vi "add scan position(SubVI).vi"(10 "字符串":string) -> (0 "布尔 3":bool, 2 "连接的字符串":string)   [LabVIEW 2019, in "SubVI.lvlib"]
uses:
  SubVI.lvlib
panel:
  in  "Number of Step":i32=2
  in  "Step Delay(secs)":dbl
  in  "Increments":dbl=10.0
  in  "cancel":bool
  in  "ok":bool
  in  "Approach":i32(ring)=1 items=["Pause", "Sweep"]
  in  "Speed":i32 min=0 max=14
  in  "Final Position":dbl min=-140000.0 max=140000.0
  in  "Initial Position":dbl min=-140000.0 max=140000.0
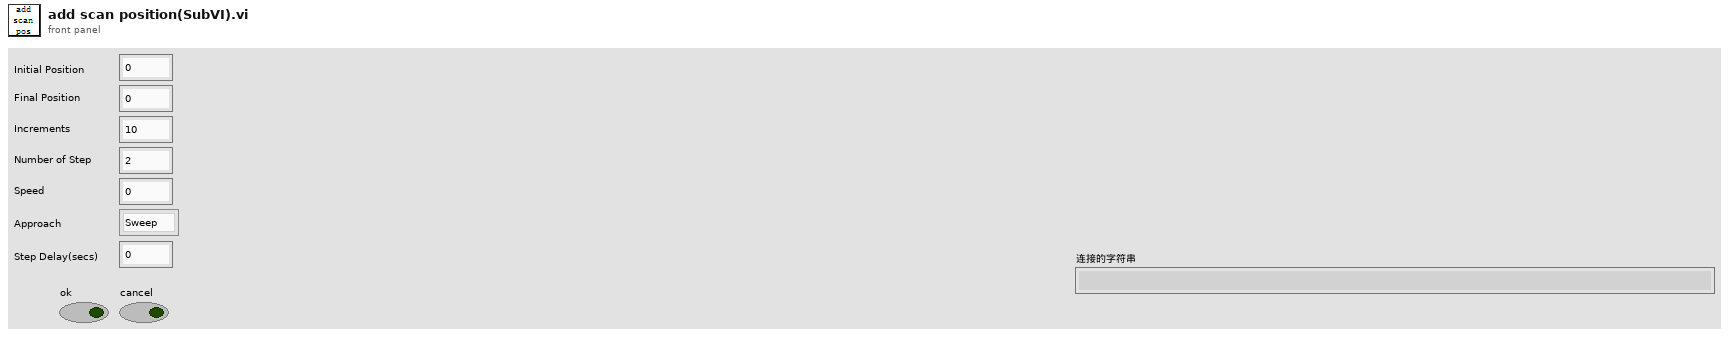
[diagram p1: front panel]
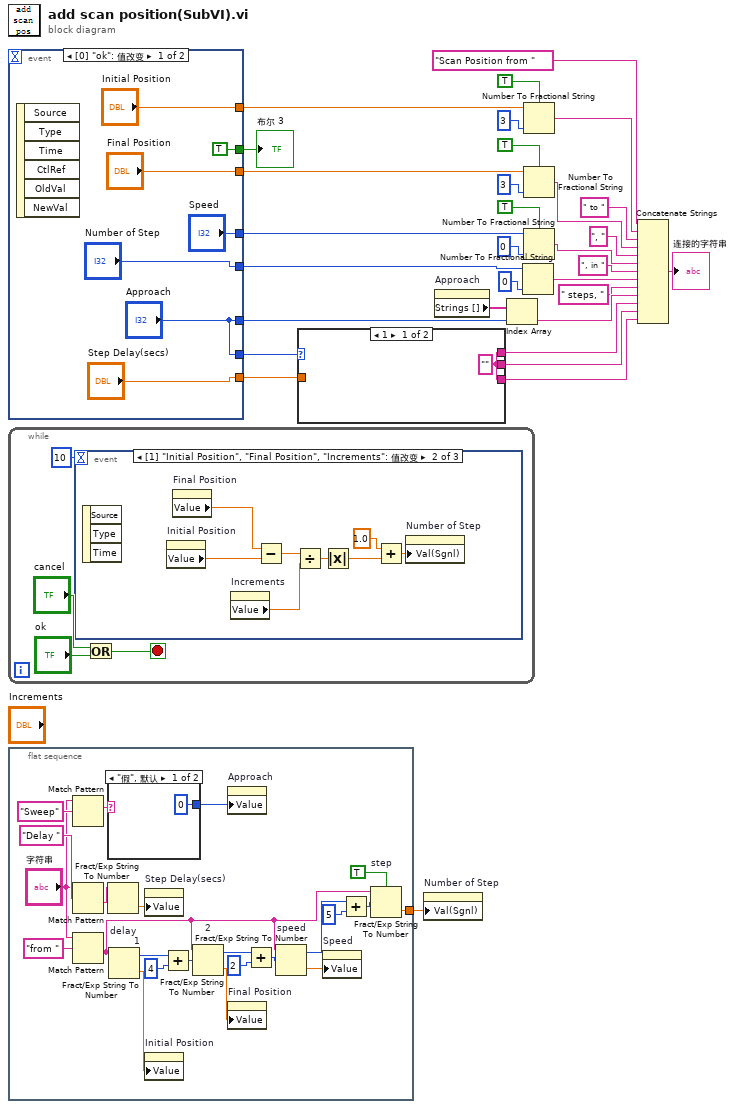
[diagram p0: block diagram]
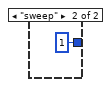
[diagram p2: hidden frame]
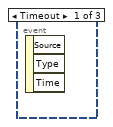
[diagram p3: hidden frame]
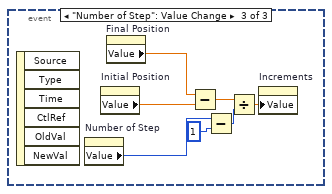
[diagram p4: hidden frame]
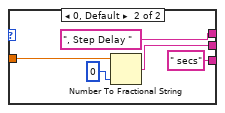
[diagram p5: hidden frame]
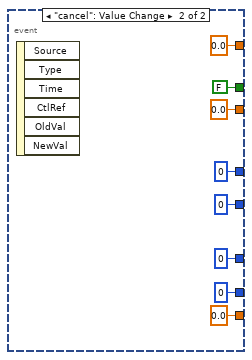
[diagram p6: hidden frame]
diagram:
  n1 = event shown="[0] \"ok\": 值改变" {
    selector: _ -> [_ _]
    dyn-events: _ -> [_ _]
    timeout: _ -> [_ _]
    tunnel: ["Final Position" 0.0 ("Field 2")] -> w20
    tunnel: ["Speed" 0 ("Rate输入")] -> w17
    tunnel: ["Initial Position" 0.0 ("Field")] -> w29
    tunnel: [TRUE FALSE] -> w31
    tunnel: ["Number of Step" 0 ("Number of Step")] -> w14
    tunnel: ["Approach" 0 ("Approach输入")] -> w10
    tunnel: ["Step Delay(secs)" 0.0 ("Step Delay(secs)")] -> w5
    tunnel: ["Approach" 0 ("Approach")] -> w3
    event "ok": Value Change {
      n2 = event-data() -> ()  [unwired: 1 in, 6 out]
    }
    event "cancel": Value Change {
      n3 = event-data() -> ()  [unwired: 1 in, 6 out]
    }
  }
  "布尔 3" <- w31
  n4 = while {
    stop <- w47 stop-if-true
    n5 = event shown="[1] \"Initial Position\", \"Final Position\", \"Increments\": 值改变" {
      selector: _ -> [_ _ _]
      dyn-events: _ -> [_ _ _]
      timeout: 10 -> [_ _ _]
      event Timeout {
        n6 = event-data() -> ()  [unwired: 1 in, 3 out]
      }
      event "Initial Position", "Final Position", "Increments": Value Change {
        n7 = event-data() -> ()  [unwired: 1 in, 3 out]
        n8 = property on="Initial Position" class="DigNum (严格)"() -> ("Value"=w57:dbl)  [unwired: 2 in, 2 out]
        n9 = property on="Final Position" class="DigNum (严格)"() -> ("Value"=w58:dbl)  [unwired: 2 in, 2 out]
        n10 = property on="Increments" class="DigNum (严格)"() -> ("Value"=w55:dbl)  [unwired: 2 in, 2 out]
        n11 = Subtract(x=w58, y=w57) -> (x-y=w56:dbl)
        n12 = Divide(x=w56, y=w55) -> (x/y=w52:dbl)
        n13 = Absolute Value(x=w52) -> (abs(x)=w51:dbl)
        n14 = Add(x=1.0, y=w51) -> (x+y=w53:dbl)
        n15 = property on="Number of Step" class="DigNum (严格)"("Val(Sgnl)"=w53) -> ()  [unwired: 2 in, 2 out]
      }
      event "Number of Step": Value Change {
        n16 = event-data() -> ()  [unwired: 1 in, 6 out]
        n17 = property on="Number of Step" class="DigNum (严格)"() -> ("Value"=w62:i32)  [unwired: 2 in, 2 out]
        n18 = property on="Initial Position" class="DigNum (严格)"() -> ("Value"=w64:dbl)  [unwired: 2 in, 2 out]
        n19 = property on="Final Position" class="DigNum (严格)"() -> ("Value"=w65:dbl)  [unwired: 2 in, 2 out]
        n20 = Subtract(x=w65, y=w64) -> (x-y=w63:dbl)
        n21 = Subtract(x=w62, y=1) -> (x-y=w60:i32)
        n22 = Divide(x=w63, y=w60) -> (x/y=w59:dbl)
        n23 = property on="Increments" class="DigNum (严格)"("Value"=w59) -> ()  [unwired: 2 in, 2 out]
      }
    }
    n24 = Or(x="cancel", y="ok") -> (x .or. y?=w47:bool)
  }
  n25 = flat-sequence {
    tunnel: [w66] -> w1
    frame #0 {
      n26 = Match Pattern(string="字符串", regular expression="Sweep" ("正则表达式")) -> (match substring=w72:string)  [unwired: 1 in, 3 out]
      n27 = Match Pattern(string="字符串", regular expression="Delay " ("正则表达式")) -> (after substring=w75:string)  [unwired: 1 in, 3 out]
      n28 = Match Pattern(string="字符串", regular expression="from " ("正则表达式")) -> (after substring=w74:string)  [unwired: 1 in, 3 out]
      n29 = case shown="\"假\", 默认" w72 {
        tunnel: [0 1] -> w71
        frame "假", Default {
        }
        frame "sweep" {
        }
      }
      n30 = Fract/Exp String To Number "delay"(string=w75) -> (number=w68:dbl)  [unwired: 3 in, 1 out]
      n31 = Fract/Exp String To Number "1"(string=w74) -> (offset past number=w87:i32, number=w69:dbl)  [unwired: 3 in]
      n32 = property on="Step Delay(secs)" class="DigNum (严格)"("Value"=w68) -> ()  [unwired: 2 in, 2 out]
      n33 = property on="Initial Position" class="DigNum (严格)"("Value"=w69) -> ()  [unwired: 2 in, 2 out]
      n34 = Add(x=w87, y=4) -> (x+y=w85:i32)
      n35 = Fract/Exp String To Number "2"(string=w74, offset=w85) -> (offset past number=w84:i32, number=w70:dbl)  [unwired: 2 in]
      n36 = property on="Approach" class="Ring (严格)"("Value"=w71) -> ()  [unwired: 2 in, 2 out]
      n37 = property on="Final Position" class="DigNum (严格)"("Value"=w70) -> ()  [unwired: 2 in, 2 out]
      n38 = Add(x=w84, y=2) -> (x+y=w82:i32)
      n39 = Fract/Exp String To Number "speed"(string=w74, offset=w82) -> (offset past number=w81:i32, number=w67:dbl)  [unwired: 2 in]
      n40 = property on="Speed" class="DigNum (严格)"("Value"=w67) -> ()  [unwired: 2 in, 2 out]
      n41 = Add(x=w81, y=5) -> (x+y=w79:i32)
      n42 = Fract/Exp String To Number "step"(use system decimal point (T)=TRUE ("使用系统小数点(T)"), string=w74, offset=w79) -> (number=w66:dbl)  [unwired: 1 in, 1 out]
    }
  }
  n43 = case shown="1" w3 {
    tunnel: [w91 ", Step Delay " ("字符串")] -> w7
    tunnel: [w91 " secs" ("字符串")] -> w6
    tunnel: w5 -> [_ w94]
    tunnel: [w91 w93] -> w4
    frame 1 {
      w91 = ""
    }
    frame 0, Default {
      n44 = Number To Fractional String(number=w94, precision (6)=i16 0 ("精度(6)")) -> (F-format string=w93:string)  [unwired: 2 in]
    }
  }
  n45 = property on="Number of Step" class="DigNum (严格)"("Val(Sgnl)"=w1) -> ()  [unwired: 2 in, 2 out]
  n46 = property on="Approach" class="Ring (严格)"() -> ("Strings []"=w11:string[])  [unwired: 2 in, 2 out]
  n47 = Index Array(array=w11, index=w10) -> (element=w8:string)
  n48 = Number To Fractional String(number=w14, precision (6)=i16 0 ("精度(6)")) -> (F-format string=w13:string)  [unwired: 2 in]
  n49 = Number To Fractional String(use system decimal point (T)=TRUE ("使用系统小数点(T)"), number=w29, precision (6)=i16 3 ("精度(6)")) -> (F-format string=w27:string)  [unwired: 1 in]
  n50 = Number To Fractional String(use system decimal point (T)=TRUE ("使用系统小数点(T)"), number=w20, precision (6)=i16 3 ("精度(6)")) -> (F-format string=w22:string)  [unwired: 1 in]
  n51 = Number To Fractional String(use system decimal point (T)=TRUE ("使用系统小数点(T)"), number=w17, precision (6)=i16 0 ("精度(6)")) -> (F-format string=w16:string)  [unwired: 1 in]
  n52 = Concatenate Strings("Scan Position from " ("字符串"), w27, " to " ("字符串"), w22, ", " ("字符串"), w16, ", in " ("字符串"), w13, " steps, " ("字符串"), w8, w7, w4, w6) -> (→"连接的字符串":string)
